vi "HitrapGUI.HTLE_NoGUI.vi"() -> ()   [LabVIEW 2014, in "HitrapGUI.lvlib"]
uses:
  HitrapGUI.lvlib
  CSlibraries/GUILib/GUILib.userEventsMainType.ctl
  CSlibraries-extern/DimLVEvent/DimIndicators/DimIndicators.anyType.ctl
  CSlibraries/GUILib/GUILib.simpleNumeric.ctl
  CSlibraries/GUILib/GUILib.basicNumeric.ctl
  CSlibraries/GUILib/GUILib.simpleBoolean.ctl
  CSlibraries/GUILib/GUILib.basicBoolean.ctl
  CSlibraries/UtilityLib/UtilityLib.valueStatus.ctl
  CS_Core/CSSystem/CoreDefs/CoreDefs.rawDataType.ctl
  CS_Core/CSSystem/CoreLib/CoreLib.double 2 byte array.vi
  CS_Core/CSSystem/CoreLib/CoreLib.short 2 byte array.vi
  CSlibraries/UtilityLib/UtilityLib.lvlib
  CS_Core/CSSystem/CSSystemLib/CSSystemLib.lvlib
  CSlibraries-extern/DimLVEvent/DimIndicators/DimIndicators.lvlib
  CS_Core/GUIs/GOGControllerGUI/GOGControllerGUI.lvlib
  CSlibraries/GUILib/GUILib.lvlib
  CS_Core/CSSystem/CoreLib/CoreLib.lvlib
panel:
  in  "digital5":bool=TRUE
  in  "digital4":bool=TRUE
  in  "digital3":bool=TRUE
  in  "digital2":bool=TRUE
  in  "digital5Ctl":T1
  in  "digital4Ctl":T1
  in  "digital3Ctl":T1
  in  "digital2Ctl":T1
  in  "digital1":bool=TRUE
  in  "digital1Ctl":T1
  in  "analog5Ctl":T3 {"nom" step=1.0}
  in  "analog5":bool=TRUE
  in  "analog4Ctl":T3 {"nom" step=1.0}
  in  "analog4":bool=TRUE
  in  "analog3Ctl":T3 {"nom" step=1.0}
  in  "analog3":bool=TRUE
  in  "analog2Ctl":T3 {"nom" step=1.0}
  in  "analog2":bool=TRUE
  in  "analog1Ctl":T3 {"nom" step=1.0}
  in  "analog1":bool=TRUE
  out "subSystem1State":string
  in  "subSystem1":bool
  out "subSystem1StateQuality":string
  in  "subControllersIgnoredDIM":T5
  in  "iniData":string
  in  "stop":bool
  in  "dummy":bool
  in  "parentSystem":bool
  in  "userEvent":refnum<user-event>
  # "NoGUI"
  # "(contains devices/elements that have no dedicated GUI yet)"
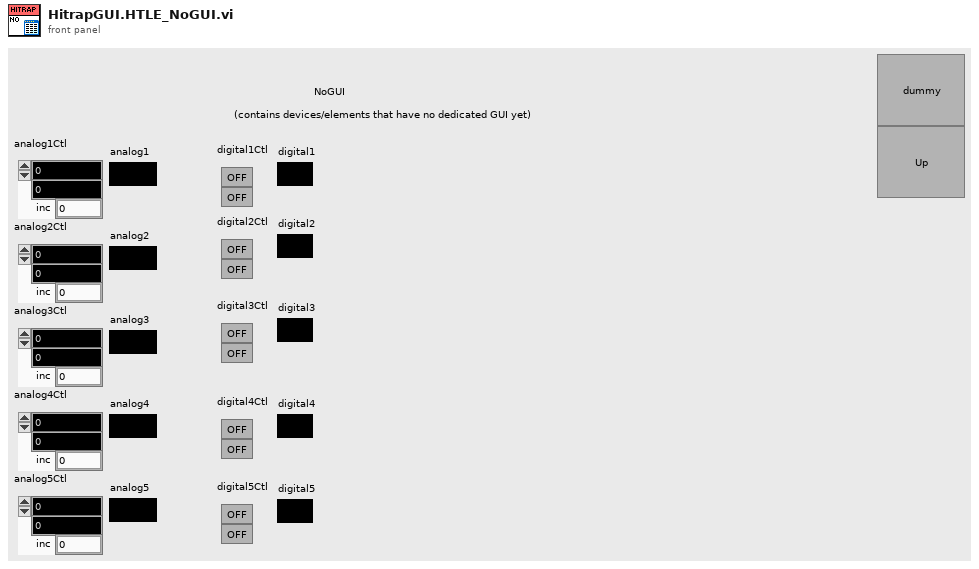
[diagram p1: front panel]
types:
  T1 = typedef "GUILib.lvlib/GUILib.simpleBoolean.ctl" = cluster{"nominal":T2, "actual":T2}
  T2 = typedef "GUILib.lvlib/GUILib.basicBoolean.ctl" = bool
  T3 = typedef "GUILib.lvlib/GUILib.simpleNumeric.ctl" = cluster{"nom":T4, "act":dbl, "inc":dbl}
  T4 = typedef "GUILib.lvlib/GUILib.basicNumeric.ctl" = dbl
  T5 = typedef "DimIndicators.lvlib/DimIndicators.anyType.ctl" = cluster{"data":string, "no link":bool, "quality":i32, "timeStamp":dbl}
  T6 = typedef "UtilityLib.lvlib/UtilityLib.valueStatus.ctl" = enum16{"no info available", "stand by/off", "on", "warning", "alarm/malfunction", "not implemented", "user action required", "important information", "system default", "control default", "indicator default", "button default"}
  T7 = typedef "CoreDefs.rawDataType.ctl" = i8[]
  T8 = typedef "lveventtype.ctl" = enum32{"Null", "Timeout", "Annotation Menu Selection", "Annotation Menu Selection?", "App Instance Close", "App Instance Close?", "Autoscale Range Change", "Bookmark Info Change", "Cell Edit", "Cell Edit?", "Cursor Grab", "Cursor Grab?", "Cursor Menu Selection", "Cursor Menu Selection?", "Cursor Move", "Cursor Release", "Data Change", "Direction Change", "Display State Change", "Drag Ended", "Drag Enter", "Drag Leave", "Drag Over", "Drag Source Update", "Drag Starting", "Drag Starting?", "Drop", "Exec State Change", "Key Down", "Key Down?", "Key Repeat", "Key Repeat?", "Key Up", "Listbox Double Click", "Menu Activation?", "Menu Selection (App)", "Menu Selection? (App)", "Menu Selection (User)", "Mouse Down", "Mouse Down?", "Mouse Enter", "Mouse Leave", "Mouse Move", "Mouse Up", "Mouse Wheel", "NI Security User Change (App)", "Pane Size", "Panel Close", "Panel Close?", "Panel Resize", "Plot Attribute Change", "Scale Range Change", "Shortcut Menu Activation?", "Shortcut Menu Selection (App)", "Shortcut Menu Selection? (App)", "Shortcut Menu Selection (User)", "Tree Double Click", "Tree Drag", "Tree Drag?", "Tree Drop", "Tree Drop?", "Tree Item Close", "Tree Item Close?", "Tree Item Open", "Tree Item Open?", "User Event", "Value Change"}
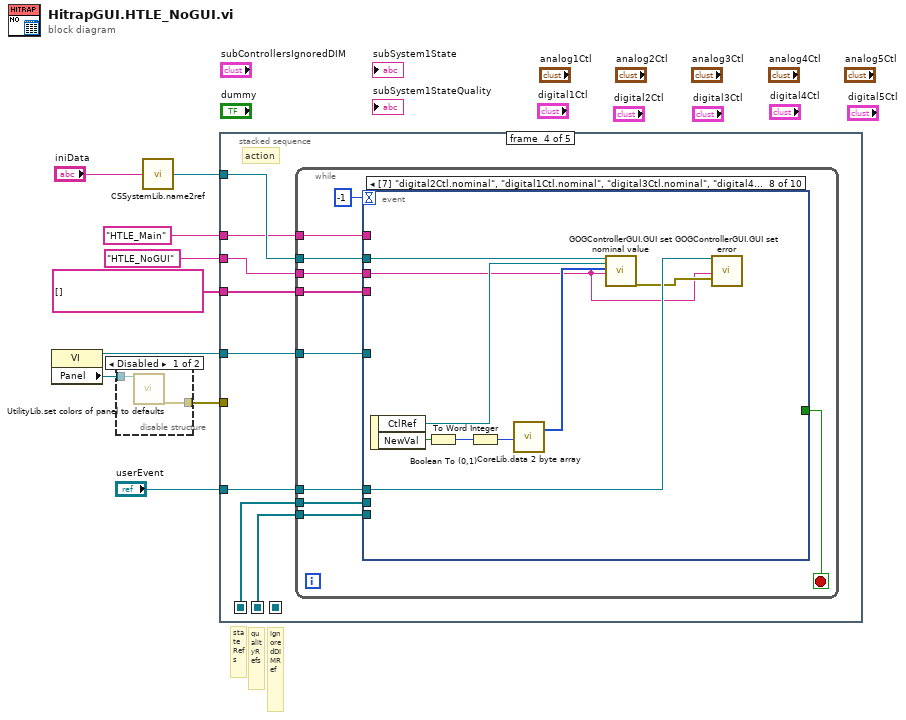
[diagram p0: block diagram]
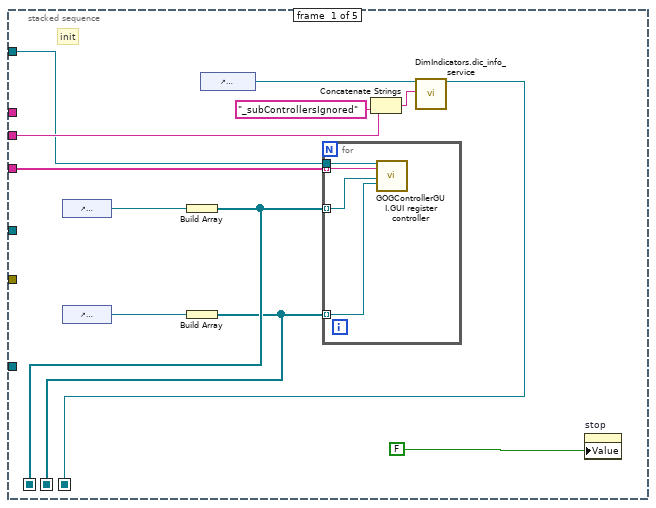
[diagram p3: hidden frame]
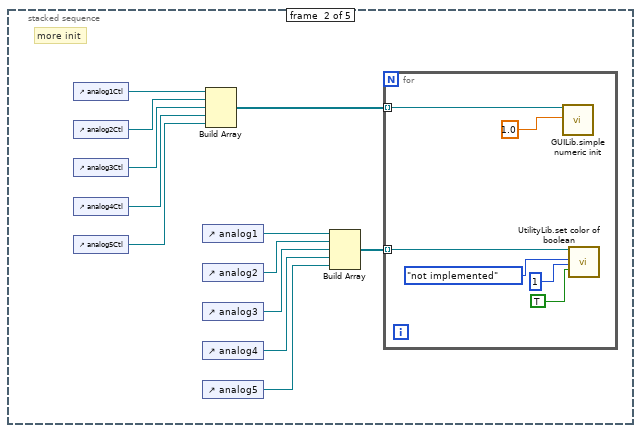
[diagram p4: hidden frame]
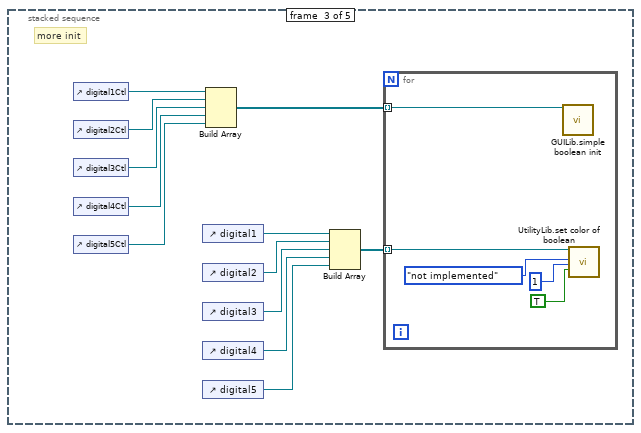
[diagram p5: hidden frame]
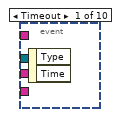
[diagram p6: hidden frame]
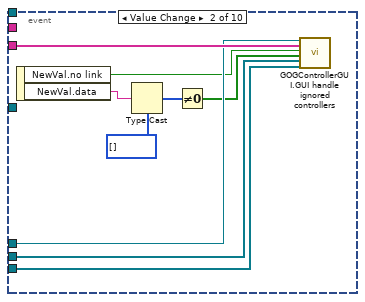
[diagram p7: hidden frame]
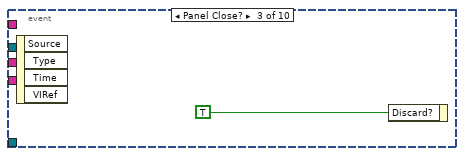
[diagram p8: hidden frame]
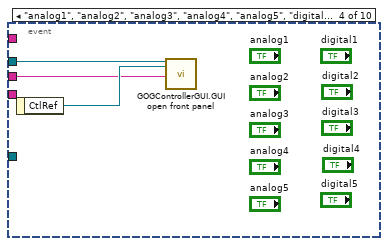
[diagram p9: hidden frame]
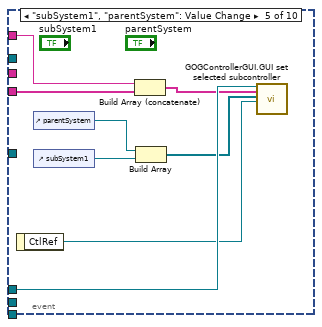
[diagram p10: hidden frame]
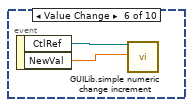
[diagram p11: hidden frame]
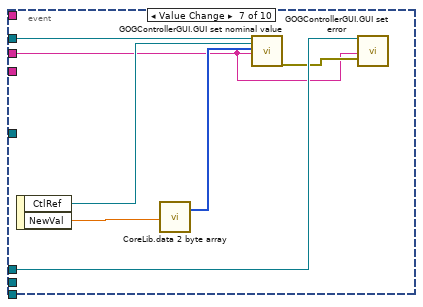
[diagram p12: hidden frame]
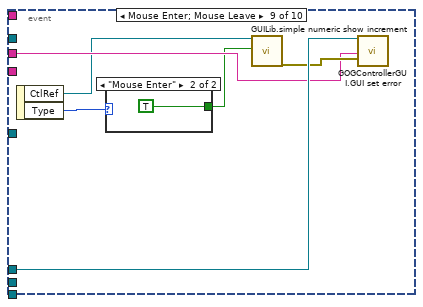
[diagram p13: hidden frame]
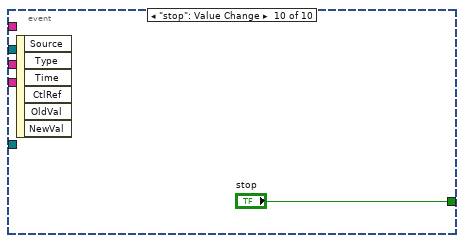
[diagram p15: hidden frame]
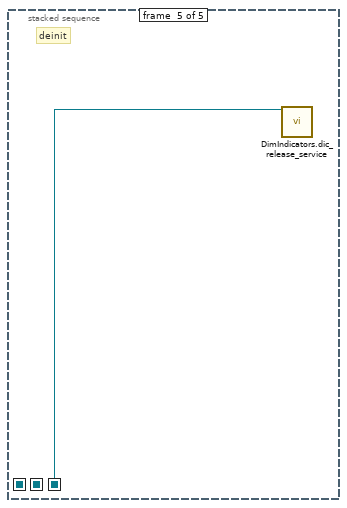
[diagram p16: hidden frame]
diagram:
  # "qualityRefs"
  # "ignoredDIMRef"
  # "stateRefs"
  n1 = property class="VI"() -> (reference out=w7:refnum<vi>, "Panel"=w8:refnum<vi>)  [unwired: 2 in, 1 out]
  n2 = disable-structure shown="Disabled" {
    disable-tunnel: w8 -> [w11 _]
    disable-tunnel: [w10 _] -> w6
    frame Disabled {
      n3 = call "UtilityLib.set colors of panel to defaults.vi"("Front Panel"=w11) -> ("error out"=w10:errorcluster)  [unwired: 18 in]
    }
    frame Enabled {
    }
  }
  n4 = call "CSSystemLib.name2ref.vi"("name"="iniData") -> ("obj refnum"=w2:refnum<vi>)
  n5 = stacked-sequence {
    seq-local: [w13 _ _ _ _] -> [_ _ _ _ w128]
    seq-local: [w14 _ _ _ _] -> [_ _ _ w67 _]
    seq-local: [w12 _ _ _ _] -> [_ _ _ w66 _]
    tunnel: "userEvent" -> [_ _ _ w70 _]
    tunnel: w7 -> [_ _ _ w69 _]
    tunnel: w6 -> [_ _ _ _ _]
    tunnel: "HTLE_NoGUI" -> [w19 _ _ w64 _]
    tunnel: string[] [] -> [w18 _ _ w68 _]
    tunnel: w2 -> [w17 _ _ w65 _]
    tunnel: "HTLE_Main" -> [_ _ _ w63 _]
    frame #0 {
      # "init"
      n6 = control-ref of="dummySubSystemState"() -> (w16:refnum<vi>)
      n7 = control-ref of="dummySubSystemStateQuality"() -> (w15:refnum<vi>)
      n8 = Build Array(w16) -> (w14:refnum<vi>[])
      n9 = Build Array(w15) -> (w12:refnum<vi>[])
      n10 = control-ref of="subControllersIgnoredDIM"() -> (w20:refnum<vi>)
      n11 = for {
        tunnel: w14 -> [w27] mode=indexing
        tunnel: w18 -> [w25] mode=indexing
        tunnel: w12 -> [w24] mode=indexing
        tunnel: w17 -> [w26]
        n12 = call "GOGControllerGUI.GUI register controller.vi"("i ref in"=w26, "controllerName"=w25, "subSystemState"=w27, "subSystemStateQuality"=w24) -> ()  [unwired: 14 in, 2 out]
      }
      n13 = Concatenate Strings(w19, "_subControllersIgnored" ("string")) -> (w22:string)
      n14 = call "DimIndicators.dic_info_service.vi"("controlRef"=w20, "serviceName"=w22) -> ("controlRef out"=w13:refnum<vi>)  [unwired: 16 in, 1 out]
      n15 = property on="stop" class="Bool (strict)"("Value"=FALSE ("stop")) -> ()  [unwired: 2 in, 2 out]
    }
    frame #1 {
      # "more init"
      n16 = control-ref of="analog1Ctl"() -> (w39:refnum<vi>)
      n17 = control-ref of="analog2Ctl"() -> (w38:refnum<vi>)
      n18 = control-ref of="analog3Ctl"() -> (w37:refnum<vi>)
      n19 = control-ref of="analog4Ctl"() -> (w36:refnum<vi>)
      n20 = control-ref of="analog5Ctl"() -> (w35:refnum<vi>)
      n21 = control-ref of="analog1"() -> (w33:refnum<vi>)
      n22 = control-ref of="analog2"() -> (w32:refnum<vi>)
      n23 = control-ref of="analog3"() -> (w31:refnum<vi>)
      n24 = control-ref of="analog4"() -> (w30:refnum<vi>)
      n25 = control-ref of="analog5"() -> (w29:refnum<vi>)
      n26 = Build Array(w39, w38, w37, w36, w35) -> (w34:refnum<vi>[])
      n27 = Build Array(w33, w32, w31, w30, w29) -> (w28:refnum<vi>[])
      n28 = for {
        tunnel: w34 -> [w45] mode=indexing
        tunnel: w28 -> [w41] mode=indexing
        n29 = call "GUILib.simple numeric init.vi"("ctlRef"=w45, "increment"=1.0) -> ()  [unwired: 16 in, 2 out]
        n30 = call "UtilityLib.set color of boolean.vi"("button"=w41, "valueStatus"=UtilityLib.valueStatus."not implemented", "nOfPair (0)"=1, "setTRUEColor (FALSE)"=TRUE) -> ()  [unwired: 15 in, 1 out]
      }
    }
    frame #2 {
      # "more init"
      n31 = control-ref of="digital1Ctl"() -> (w57:refnum<vi>)
      n32 = control-ref of="digital2Ctl"() -> (w56:refnum<vi>)
      n33 = control-ref of="digital3Ctl"() -> (w55:refnum<vi>)
      n34 = control-ref of="digital4Ctl"() -> (w54:refnum<vi>)
      n35 = control-ref of="digital5Ctl"() -> (w53:refnum<vi>)
      n36 = control-ref of="digital1"() -> (w51:refnum<vi>)
      n37 = control-ref of="digital2"() -> (w50:refnum<vi>)
      n38 = control-ref of="digital3"() -> (w49:refnum<vi>)
      n39 = control-ref of="digital4"() -> (w48:refnum<vi>)
      n40 = control-ref of="digital5"() -> (w47:refnum<vi>)
      n41 = Build Array(w57, w56, w55, w54, w53) -> (w52:refnum<vi>[])
      n42 = Build Array(w51, w50, w49, w48, w47) -> (w46:refnum<vi>[])
      n43 = for {
        tunnel: w52 -> [w62] mode=indexing
        tunnel: w46 -> [w58] mode=indexing
        n44 = call "GUILib.simple boolean init.vi"("ctlRef"=w62) -> ()  [unwired: 17 in, 2 out]
        n45 = call "UtilityLib.set color of boolean.vi"("button"=w58, "valueStatus"=UtilityLib.valueStatus."not implemented", "nOfPair (0)"=1, "setTRUEColor (FALSE)"=TRUE) -> ()  [unwired: 15 in, 1 out]
      }
    }
    frame #3 {
      # "action"
      n46 = while {
        tunnel: w70 -> [w80]
        tunnel: w69 -> [w78]
        tunnel: w68 -> [w76]
        tunnel: w67 -> [w75]
        tunnel: w66 -> [w74]
        tunnel: w65 -> [w73]
        tunnel: w64 -> [w72]
        tunnel: w63 -> [w71]
        stop <- w77 stop-if-true
        n47 = event shown="[7] \"digital2Ctl.nominal\", \"digital1Ctl.nominal\", \"digital3Ctl.nominal\", \"digital4Ctl.nominal\", \"digital5Ctl.nominal\": Value Change" {
          selector: _ -> [_ _ _ _ _ _ _ _ _ _]
          dyn-events: _ -> [_ _ _ _ _ _ _ _ _ _]
          timeout: -1 -> [_ _ _ _ _ _ _ _ _ _]
          tunnel: w80 -> [_ w85 _ _ w100 _ w106 w115 w125 _]
          tunnel: w78 -> [_ _ _ _ _ _ _ _ _ _]
          tunnel: [_ _ _ _ _ _ _ _ _ "stop"] -> w77
          tunnel: w76 -> [_ w86 _ _ w96 _ _ _ _ _]
          tunnel: w75 -> [_ w82 _ _ _ _ _ _ _ _]
          tunnel: w74 -> [_ w81 _ _ _ _ _ _ _ _]
          tunnel: w73 -> [_ _ _ w93 _ _ w110 w119 _ _]
          tunnel: w72 -> [_ _ _ w91 _ _ w104 w113 w123 _]
          tunnel: w71 -> [_ _ _ _ w95 _ _ _ _ _]
          event Timeout {
            n48 = event-data() -> ()  [unwired: 1 in, 2 out]
          }
          event Value Change {
            n49 = event-data() -> ("NewVal.no link"=w84:bool, "NewVal.data"=w87:string)  [unwired: 1 in]
            n50 = Type Cast(type=T7 [] ("Array"), x=w87) -> (*(type *) &x=w89:T7)
            n51 = Not Equal To 0?(x=w89) -> (x != 0?=w83:bool[])
            n52 = call "GOGControllerGUI.GUI handle ignored controllers.vi"("userEvent"=w85, "controllerNames"=w86, "NOLINK"=w84, "controllersIgnored"=w83, "stateRefs"=w82, "qualityRefs"=w81) -> ()  [unwired: 14 in]
          }
          event Panel Close? {
            n53 = event-data() -> ()  [unwired: 1 in, 4 out]
            n54 = event-data("Discard?"=TRUE) -> ()  [unwired: 1 in, 1 out]
          }
          event "analog1", "analog2", "analog3", "analog4", "analog5", "digital1", "digital2", "digital3", "digital4", "digital5": Value Change {
            n55 = event-data() -> ("CtlRef"=w92:refnum<vi>)  [unwired: 1 in]
            n56 = call "GOGControllerGUI.GUI open front panel.vi"("i ref in"=w93, "elementRef"=w92, "controller"=w91) -> ()  [unwired: 15 in, 2 out]
          }
          event "subSystem1", "parentSystem": Value Change {
            n57 = event-data() -> ("CtlRef"=w98:refnum<vi>)  [unwired: 1 in]
            n58 = control-ref of="parentSystem"() -> (w97:refnum<vi>)
            n59 = control-ref of="subSystem1"() -> (w101:refnum<vi>)
            n60 = Build Array (concatenate)(w95, w96) -> (w94:string[])
            n61 = Build Array(w97, w101) -> (w99:refnum<vi>[])
            n62 = call "GOGControllerGUI.GUI set selected subcontroller.vi"("userEvent"=w100, "controllerNames"=w94, "controllerRefs"=w99, "controllerRef"=w98) -> ()  [unwired: 16 in]
          }
          event Value Change {
            n63 = event-data() -> ("CtlRef"=w103:refnum<vi>, "NewVal"=w102:dbl)  [unwired: 1 in]
            n64 = call "GUILib.simple numeric change increment.vi"("ctlRef"=w103, "increment"=w102) -> ()  [unwired: 16 in, 2 out]
          }
          event Value Change {
            n65 = event-data() -> ("CtlRef"=w109:refnum<vi>, "NewVal"=w108:T4)  [unwired: 1 in]
            n66 = call-poly "CoreLib.data 2 byte array.vi"("f64"=w108) -> ("byteArray out"=w107:T7)  [unwired: 18 in]
            n67 = call "GOGControllerGUI.GUI set nominal value.vi"("i ref in"=w110, "nominalRef"=w109, "nominalData"=w107, "controller"=w104) -> ("error out"=w105:errorcluster)  [unwired: 14 in, 1 out]
            n68 = call "GOGControllerGUI.GUI set error.vi"("userEvent"=w106, "controller"=w104, "GUIError"=w105) -> ()  [unwired: 16 in, 1 out]
          }
          event Value Change {
            n69 = event-data() -> ("CtlRef"=w118:refnum<vi>, "NewVal"=w117:T2)  [unwired: 1 in]
            n70 = Boolean To (0,1)(Boolean=w117) -> (0, 1=w112:i16)
            n71 = To Word Integer(number=w112) -> (16bit integer=w111:i16)
            n72 = call-poly "CoreLib.data 2 byte array.vi"("i16"=w111) -> ("byteArray out"=w116:T7)  [unwired: 18 in]
            n73 = call "GOGControllerGUI.GUI set nominal value.vi"("i ref in"=w119, "nominalRef"=w118, "nominalData"=w116, "controller"=w113) -> ("error out"=w114:errorcluster)  [unwired: 14 in, 1 out]
            n74 = call "GOGControllerGUI.GUI set error.vi"("userEvent"=w115, "controller"=w113, "GUIError"=w114) -> ()  [unwired: 16 in, 1 out]
          }
          event Mouse Enter; Mouse Leave {
            n75 = event-data() -> ("CtlRef"=w122:refnum<vi>, "Type"=w121:T8)  [unwired: 1 in]
            n76 = case shown="\"Mouse Enter\"" w121 {
              tunnel: [_ TRUE] -> w120
              frame Default {
              }
              frame "Mouse Enter" {
              }
            }
            n77 = call "GUILib.simple numeric show increment.vi"("ctlRef"=w122, "show"=w120) -> ("error out"=w124:errorcluster)  [unwired: 16 in, 1 out]
            n78 = call "GOGControllerGUI.GUI set error.vi"("userEvent"=w125, "controller"=w123, "GUIError"=w124) -> ()  [unwired: 16 in, 1 out]
          }
          event "stop": Value Change {
            n79 = event-data() -> ()  [unwired: 1 in, 6 out]
          }
        }
      }
    }
    frame #4 {
      # "deinit"
      n80 = call "DimIndicators.dic_release_service.vi"("controlRef"=w128) -> ()  [unwired: 18 in, 1 out]
    }
  }
